vi "verify #cycles.vi"(8 "error in (no error)":errorcluster, 11 "Channel in":refnum<class "Channel.lvclass">) -> (0 "error out":errorcluster, 3 "Channel out":refnum<class "Channel.lvclass">)   [LabVIEW 2018, in "Channel.lvclass"]
uses:
  Channel.lvclass
  Channel.lvclass/Channel.ctl
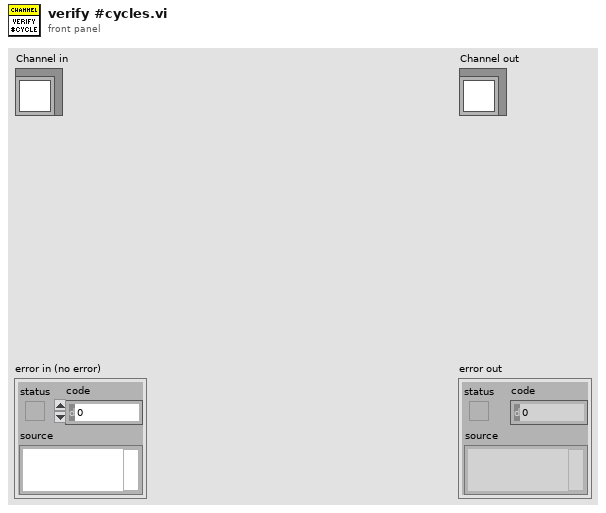
[diagram p1: front panel]
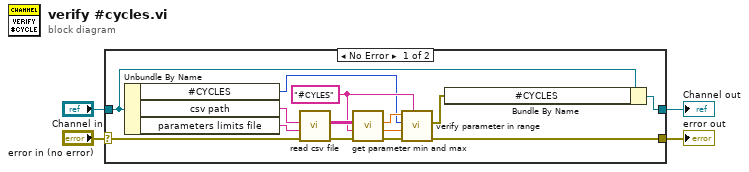
[diagram p0: block diagram]
diagram:
  n1 = case shown="No Error" "error in (no error)" {
    selector: "error in (no error)" -> [w17 w20]
    tunnel: [w10 w20] -> w3
    tunnel: [w8 w19] -> w1
    tunnel: "Channel in" -> [w9 w19]
    frame No Error {
      w11 = "#CYLES" ("parameter name")
      n2 = Unbundle By Name(w9) -> ("#CYCLES"=w5:u32, "csv path"=w18:string, "parameters limits file"=w6:string)
      n3 = call "read csv file.vi"("error in"=w17, "file name"=w6, "file path"=w18) -> ("error out"=w15:errorcluster, "csv array"=w16:string[][])  [unwired: 7 in]
      n4 = call "get parameter min and max.vi"("error in (no error)"=w15, "parameter name"=w11, "limit values"=w16) -> ("error out"=w14:errorcluster, "min"=w13:dbl, "max"=w12:dbl)  [unwired: 6 in]
      n5 = call "verify parameter in range.vi"("parameter name"=w11, "error in (no error)"=w14, "lower limit"=w13, "value"=w5, "upper limit"=w12) -> ("error out"=w10:errorcluster, "verific error"=w7:errorcluster)  [unwired: 5 in]
      n6 = Bundle By Name(cluster=w9, "#CYCLES"=w7) -> (w8:refnum<class "Channel.lvclass">)
    }
    frame Error {
    }
  }
  "error out" <- w3
  "Channel out" <- w1
